vi "load_data.vi"(8 "error in (no error)":errorcluster) -> (0 "error out":errorcluster, 1 "cancelled?":bool, 2 "position feedback":T1, 3 "ImageCollection.lvclass":refnum<class "ImageCollection.lvclass">)   [LabVIEW 2010]
uses:
  common/classes/ImageCollection/ImageCollection/position_channels_cluster.ctl
  common/classes/ImageCollection/ImageCollection/ImageCollection.lvclass
  common/classes/ImageCollection/ImageCollection/storage_mode_enum.ctl
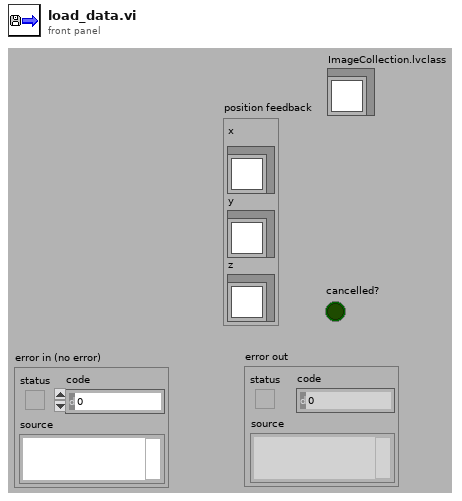
[diagram p1: front panel]
types:
  T1 = typedef "ImageCollection.lvclass/position_channels_cluster.ctl" = cluster{"x":refnum<class "ImageCollection.lvclass">, "y":refnum<class "ImageCollection.lvclass">, "z":refnum<class "ImageCollection.lvclass">}
  T2 = typedef "ImageCollection.lvclass/storage_mode_enum.ctl" = enum16{"RAM", "single files", "multipage TIFF (read-only)"}
  T3 = typedef "Image Type" = u32
  T4 = cluster{"[0]":refnum<class "ImageCollection.lvclass">, "[1]":refnum<class "ImageCollection.lvclass">, "[2]":refnum<class "ImageCollection.lvclass">}
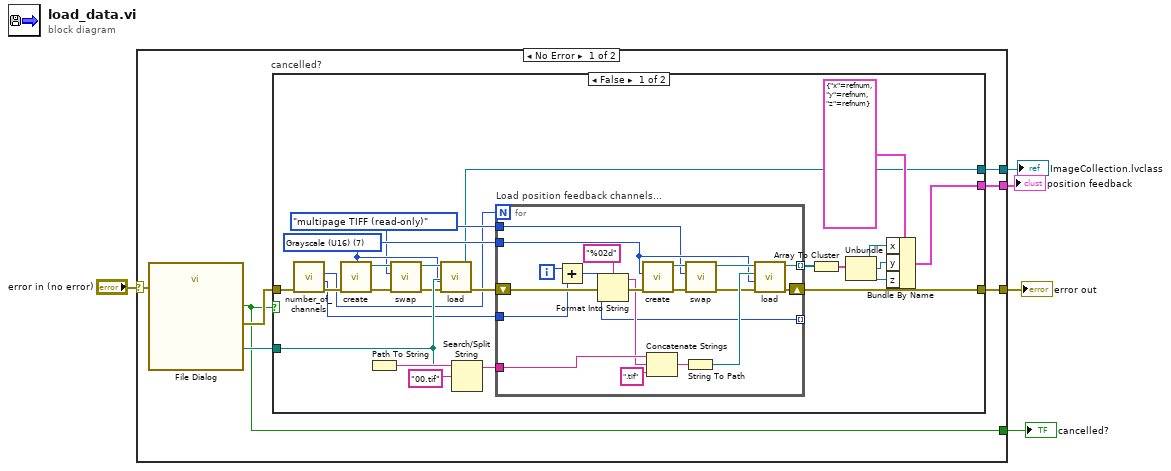
[diagram p0: block diagram]
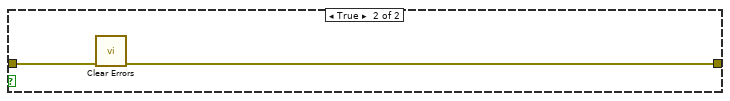
[diagram p2: hidden frame]
diagram:
  n1 = case shown="No Error" "error in (no error)" {
    selector: "error in (no error)" -> [w9 w58]
    tunnel: [w10 w58] -> w5
    tunnel: [w8 _] -> w3
    tunnel: [w7 _] -> w2
    tunnel: [w6 _] -> w1
    frame No Error {
      n2 = call "File Dialog"("error in"=w9) -> ("selected path"=w11:path, "cancelled"=w6:bool, "error out"=w12:errorcluster)  [unwired: 11 in, 1 out]
      n3 = case "cancelled?" shown="False" w6 {
        tunnel: w12 -> [w16 w57]
        tunnel: [w19 w56] -> w10
        tunnel: [w17 _] -> w7
        tunnel: w11 -> [w34 _]
        tunnel: [w33 _] -> w8
        frame False {
          w21 = storage_mode_enum."multipage TIFF (read-only)" ("target storage mode")
          w22 = T3 7 items=["Grayscale (U8)", "Grayscale (I16)", "Grayscale (SGL)", "Complex (CSG)", "RGB (U32)", "HSL (U32)", "RGB (U64)", "Grayscale (U16)"] ("Image Type")
          n4 = call "number_of_channels.vi"("error in (no error)"=w16) -> ("error IO"=w15:errorcluster, "Number of colour channels"=w14:i32, "Number of position channels"=w13:i32)  [unwired: 8 in]
          n5 = call "create.vi"("error in (no error)"=w15, "Image Type"=w22) -> ("error out"=w31:errorcluster, "ImageCollection out"=w32:refnum<class "ImageCollection.lvclass">)  [unwired: 8 in]
          n6 = Path To String(path=w34) -> (string=w35:string)
          n7 = call-dynamic "swap.vi"("error in (no error)"=w31, "target storage mode"=w21, "ImageCollection in"=w32) -> ("error out"=w30:errorcluster, "ImageCollection out"=w29:refnum<class "ImageCollection.lvclass">)  [unwired: 6 in, 1 out]
          n8 = call "load.vi"("error in (no error)"=w30, "Image Type"=w22, "path in"=w34, "ImageCollection in"=w29) -> ("error out"=w18:errorcluster, "ImageCollection out"=w17:refnum<class "ImageCollection.lvclass">)  [unwired: 3 in, 3 out]
          n9 = Search/Split String(string=w35, search string/char (-)="00.tif") -> (substring before match=w28:string)  [unwired: 1 in, 2 out]
          n10 = for "Load position feedback channels..." {
            N: w13 -> [_]
            tunnel: [w55] -> w27 mode=indexing
            shift-right: [w54] -> w19
            shift-left: w18 -> [w43]
            tunnel: w28 -> [w41]
            tunnel: w22 -> [w46]
            tunnel: w21 -> [w45]
            tunnel: [w38] -> _ mode=indexing
            tunnel: w14 -> [w37]
            i -> [w44]
            n11 = Add(x=w44, y=w37) -> (x+y=w38:i32)
            n12 = Format Into String(format string="%02d", error in=w43, w38) -> (resulting string=w40:string, error out=w42:errorcluster)  [unwired: 1 in]
            n13 = call "create.vi"("error in (no error)"=w42, "Image Type"=w46) -> ("error out"=w47:errorcluster, "ImageCollection out"=w50:refnum<class "ImageCollection.lvclass">)  [unwired: 8 in]
            n14 = Concatenate Strings(w41, w40, ".tif" ("string")) -> (w53:string)
            n15 = String To Path(string=w53) -> (path=w51:path)
            n16 = call-dynamic "swap.vi"("error in (no error)"=w47, "target storage mode"=w45, "ImageCollection in"=w50) -> ("error out"=w49:errorcluster, "ImageCollection out"=w48:refnum<class "ImageCollection.lvclass">)  [unwired: 6 in, 1 out]
            n17 = call "load.vi"("error in (no error)"=w49, "Image Type"=w46, "path in"=w51, "ImageCollection in"=w48) -> ("error out"=w54:errorcluster, "ImageCollection out"=w55:refnum<class "ImageCollection.lvclass">)  [unwired: 3 in, 3 out]
          }
          n18 = Array To Cluster(array=w27) -> (cluster=w26:T4)
          n19 = Unbundle(w26) -> ("[0]"=w25:refnum<class "ImageCollection.lvclass">, "[1]"=w24:refnum<class "ImageCollection.lvclass">, "[2]"=w23:refnum<class "ImageCollection.lvclass">)
          n20 = Bundle By Name(cluster=T1 {"x"=refnum, "y"=refnum, "z"=refnum} ("position feedback"), "x"=w25, "y"=w24, "z"=w23) -> (w33:T1)
        }
        frame True {
          n21 = call <vilib>:"Clear Errors.vi"("error in (no error)"=w57) -> ("error out"=w56:errorcluster)  [unwired: 6 in]
        }
      }
    }
    frame Error {
    }
  }
  "error out" <- w5
  "position feedback" <- w3
  "ImageCollection.lvclass" <- w2
  "cancelled?" <- w1
